vi "DeInit.vi"(8 "error in":errorcluster, 11 "Plugin_Driver in":refnum<class "Plugin_Driver.lvclass">) -> (0 "error out":errorcluster, 3 "Plugin_Driver out":refnum<class "Plugin_Driver.lvclass">)   [LabVIEW 2020, in "Plugin.lvlib" / "Plugin_Driver.lvclass"]
doc: "This VI is a wrapper API for Instrument Driver's Close API."
uses:
  Plugin_Driver.lvclass
  Drivers/Instrument Driver/Instrument Driver.lvclass
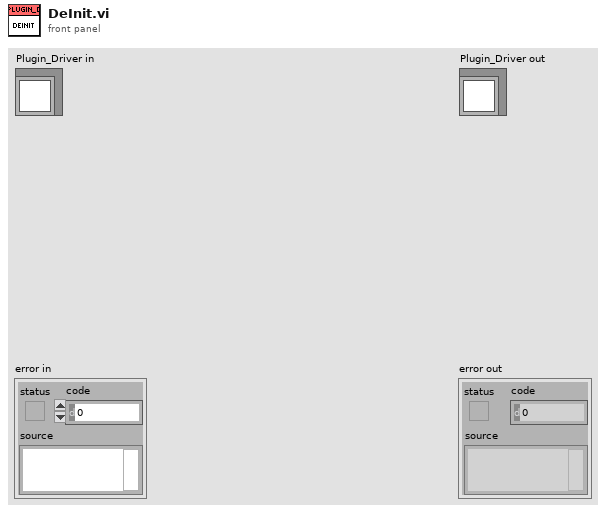
[diagram p1: front panel]
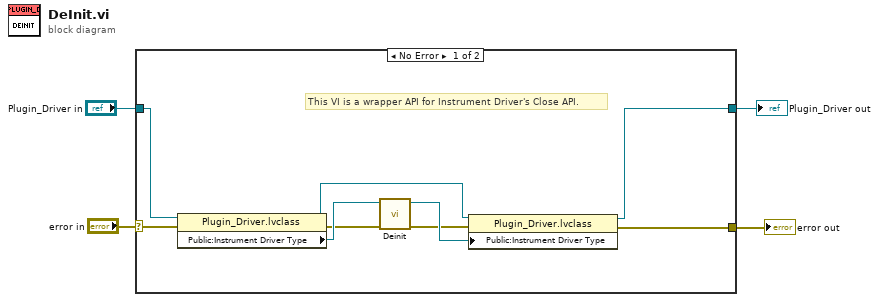
[diagram p0: block diagram]
diagram:
  n1 = case shown="No Error" "error in" {
    selector: "error in" -> [w6 w15]
    tunnel: [w8 w15] -> w3
    tunnel: [w7 w14] -> w1
    tunnel: "Plugin_Driver in" -> [w13 w14]
    frame No Error {
      # "This VI is a wrapper API for Instrument Driver's Close API."
      n2 = property class="Plugin_Driver.lvclass"(reference=w13, error in=w6) -> (reference out=w11:refnum<class "Plugin_Driver.lvclass">, error out=w5:errorcluster, "Public:Instrument Driver Type"=w12:refnum<class "Instrument Driver.lvclass">)
      n3 = call-dynamic "Deinit.vi"("error in"=w5, "Instrument Driver in"=w12) -> ("error out"=w9:errorcluster, "Instrument Driver out"=w10:refnum<class "Instrument Driver.lvclass">)  [unwired: 8 in]
      n4 = property class="Plugin_Driver.lvclass"(reference=w11, error in=w9, "Public:Instrument Driver Type"=w10) -> (reference out=w7:refnum<class "Plugin_Driver.lvclass">, error out=w8:errorcluster)
    }
    frame Error {
    }
  }
  "error out" <- w3
  "Plugin_Driver out" <- w1
